vi "Benchmark muParser_SubVI.vi"(8 "error in (no error)":errorcluster, 10 "Iterations":i32, 11 "Expression":string) -> (0 "error out":errorcluster, 2 "x":dbl[](array[numeric]), 3 "y":dbl[](array[numeric]), 5 "dt":u32)   [LabVIEW 2015]
uses:
  muExpr/muExpr.lvclass/muExpr.ctl
  muExpr/Eval.vi
  mupLib/mupSetVarValue.vi
  mupLib/mupEval.vi
  mupLib/mupCheckError.vi
  <vilib>/Utility/error.llb/Error Cluster From Error Code.vi
  muExpr/muExpr.lvclass
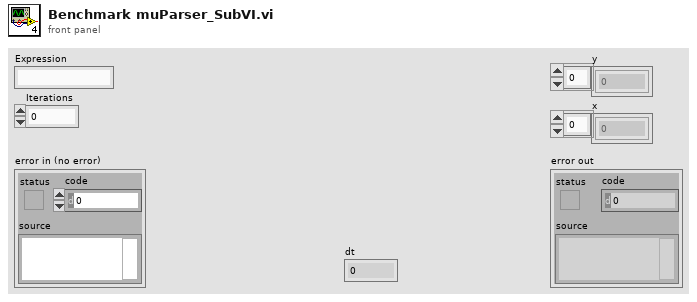
[diagram p1: front panel]
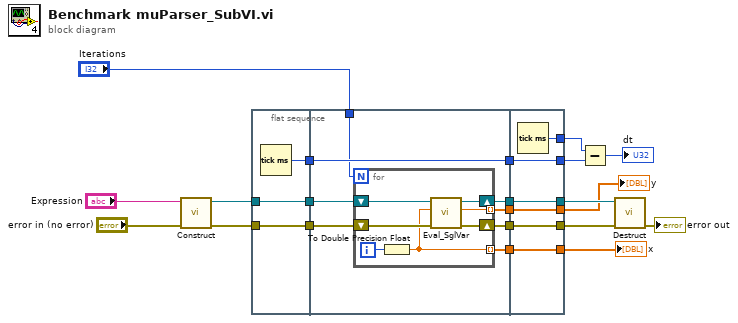
[diagram p0: block diagram]
diagram:
  n1 = call "Construct.vi"("error in (no error)"="error in (no error)", "Expression"="Expression") -> ("error out"=w19:errorcluster, "muExpr out"=w20:refnum<class "muExpr.lvclass">)  [unwired: 7 in, 1 out]
  n2 = flat-sequence {
    tunnel: w19 -> [w23]
    tunnel: w20 -> [w24]
    tunnel: [w24] -> w12
    tunnel: [w23] -> w11
    tunnel: [w22] -> w5
    tunnel: w12 -> [w32]
    tunnel: w11 -> [w31]
    tunnel: [w30] -> w10
    tunnel: [w29] -> w9
    tunnel: [w28] -> w8
    tunnel: [w27] -> w7
    tunnel: [w26] -> w6
    tunnel: w5 -> [w26]
    tunnel: "Iterations" -> [w25]
    tunnel: [w42] -> w15
    tunnel: [w43] -> w16
    tunnel: [w44] -> w17
    tunnel: [w45] -> w18
    tunnel: w10 -> [w45]
    tunnel: w9 -> [w44]
    tunnel: w8 -> [w43]
    tunnel: w7 -> [w42]
    tunnel: [w41] -> w3
    tunnel: w6 -> [w41]
    tunnel: [w40] -> w4
    frame #0 {
      n3 = Tick Count (ms)() -> (millisecond timer value=w22:u32)
    }
    frame #1 {
      n4 = for {
        N: w25 -> [_]
        shift-right: [w37] -> w29
        shift-left: w31 -> [w38]
        shift-right: [w36] -> w30
        shift-left: w32 -> [w35]
        tunnel: [w33] -> w28 mode=indexing
        tunnel: [w34] -> w27 mode=indexing
        i -> [w39]
        n5 = To Double Precision Float(number=w39) -> (double precision float=w34:dbl)
        n6 = call "Eval_SglVar.vi"("error in (no error)"=w38, "varValue"=w34, "muExpr in"=w35) -> ("error out"=w37:errorcluster, "Result"=w33:dbl, "muExpr out"=w36:refnum<class "muExpr.lvclass">)  [unwired: 6 in]
      }
    }
    frame #2 {
      n7 = Tick Count (ms)() -> (millisecond timer value=w40:u32)
    }
  }
  n8 = Subtract(x=w4, y=w3) -> (x-y=→"dt":u32)
  n9 = call "Destruct.vi"("error in (no error)"=w17, "muExpr in"=w18) -> ("error out"=→"error out":errorcluster)  [unwired: 9 in]
  "y" <- w16
  "x" <- w15
